vi "putHardpointStatus.vi"(8 "error in (no error)":errorcluster, 10 "TelemetryHardpointStatus":T1, 11 "M1M3SAL in":refnum<class "M1M3SAL.lvclass">) -> (0 "error out":errorcluster, 3 "M1M3SAL out":refnum<class "M1M3SAL.lvclass">)   [LabVIEW 2016, in "M1M3SupportCommunicator.lvlib" / "M1M3SAL.lvclass"]
uses:
  M1M3SAL.lvclass
  DataTypes/Topics/TelemetryHardpointStatus.ctl
  DataTypes/Topics/Parts/Timestamp.ctl
  DataTypes/MessageHeader.ctl
  DataTypes/MessageTypes.ctl
  DataTypes/MessageTopics.ctl
  M1M3SAL.lvclass/M1M3SAL.ctl
  writeU8.vi
  writeI32.vi
  writeBoolean.vi
  M1M3SupportCommunicator.lvlib
  DataTypes/Topics/M1M3SupportTopics.lvlib
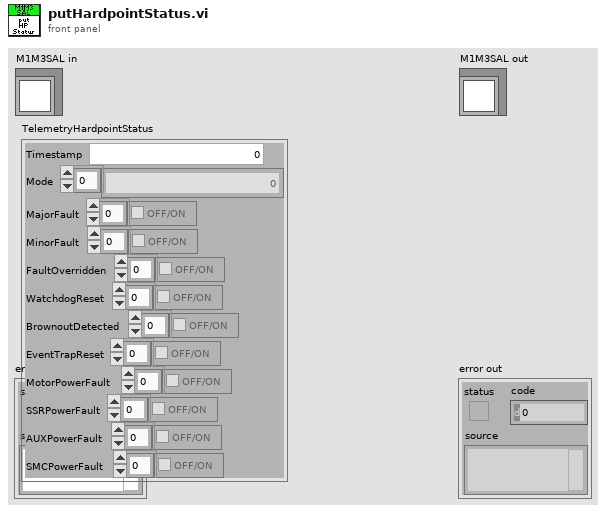
[diagram p1: front panel]
types:
  T1 = typedef "M1M3SupportTopics.lvlib/TelemetryHardpointStatus.ctl" = cluster{"Timestamp":T2, "Mode":u8[], "MajorFault":bool[], "MinorFault":bool[], "FaultOverridden":bool[], "WatchdogReset":bool[], "BrownoutDetected":bool[], "EventTrapReset":bool[], "MotorPowerFault":bool[], "SSRPowerFault":bool[], "AUXPowerFault":bool[], "SMCPowerFault":bool[]}
  T2 = typedef "M1M3SupportTopics.lvlib/Timestamp.ctl" = dbl
  T3 = typedef "M1M3SupportCommunicator.lvlib/MessageHeader.ctl" = cluster{"Type":T4, "Topic":T5, "Size":i32}
  T4 = typedef "M1M3SupportCommunicator.lvlib/MessageTypes.ctl" = enum8{"None", "PutSample", "GetNextSample", "LogEvent", "GetEvent", "IssueCommand", "CommandId", "WaitForCompletion", "AcceptCommand", "AckCommand"}
  T5 = typedef "M1M3SupportCommunicator.lvlib/MessageTopics.ctl" = enum8{"None", "ForceActuatorData", "MirrorForceData", "HardpointData", "AirData", "DynamicData", "FPGAData", "IMSData", "ForceActuatorStatus", "ElevationData", "HardpointStatus", "HardpointActuatorChase", "AirStatus", "ForceActuatorSafetyChecks", "ForceActuatorTest", "ActuatorBroadcastCounter", "StatusChecks", "CellChecks", "HardpointActuatorBreakaway", "RaiseMirrorComplete", "ILCCommunication", "ElevationAngleChecks", "DetailedState", "ServoLoops", "ForceActuatorInfo", "LowerMirrorComplete", "HardpointActuatorInfo", "SettingsApplied", "ErrorCode", "StartupChecks", "SummaryState", "SettingVersions", "ActuatorTestStatus", "AppliedSettingsMatchStart", "Enable", "EnterMaintenance", "Standby", "AbortLowerM1M3", "ApplyAberrationByForces", "ApplyAOSCorrectionByBendingModes", "ClearAOSCorrection", "Start", "RaiseM1M3", "TestForceActuator", "LowerM1M3", "ApplyAOSCorrectionByForces", "Disable", "ApplyAberationByBendingMode", "TestHardpoint", "ManipulateM1M3", "ClearAberration", "Exit", "TestAir", "AbortRaiseM1M3", "MoveHardpointActuators", "ExitMaintenance", "Shutdown"}
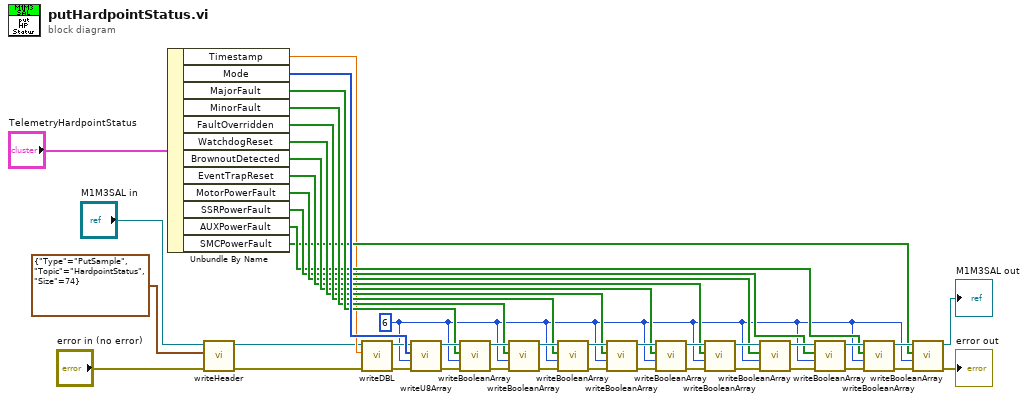
[diagram p0: block diagram]
diagram:
  w2 = 6 ("Length")
  n1 = Unbundle By Name("TelemetryHardpointStatus") -> ("Timestamp"=w9:T2, "Mode"=w20:u8[], "MajorFault"=w19:bool[], "MinorFault"=w18:bool[], "FaultOverridden"=w17:bool[], "WatchdogReset"=w16:bool[], "BrownoutDetected"=w15:bool[], "EventTrapReset"=w14:bool[], "MotorPowerFault"=w13:bool[], "SSRPowerFault"=w12:bool[], "AUXPowerFault"=w11:bool[], "SMCPowerFault"=w10:bool[])
  n2 = call "writeHeader.vi"("error in (no error)"="error in (no error)", "MessageHeader"=T3 {"Type"=enum."PutSample", "Topic"=enum."HardpointStatus", "Size"=74}, "M1M3SAL in"="M1M3SAL in") -> ("error out"=w5:errorcluster, "M1M3SAL out"=w6:refnum<class "M1M3SAL.lvclass">)  [unwired: 7 in]
  n3 = call "writeDBL.vi"("error in (no error)"=w5, "Input"=w9, "M1M3SAL in"=w6) -> ("error out"=w7:errorcluster, "M1M3SAL out"=w8:refnum<class "M1M3SAL.lvclass">)  [unwired: 7 in]
  n4 = call "writeU8Array.vi"("error in (no error)"=w7, "Length"=w2, "Input"=w20, "M1M3SAL in"=w8) -> ("error out"=w21:errorcluster, "M1M3SAL out"=w22:refnum<class "M1M3SAL.lvclass">)  [unwired: 6 in]
  n5 = call "writeBooleanArray.vi"("error in (no error)"=w21, "Length"=w2, "Input"=w19, "M1M3SAL in"=w22) -> ("error out"=w40:errorcluster, "M1M3SAL out"=w39:refnum<class "M1M3SAL.lvclass">)  [unwired: 6 in]
  n6 = call "writeBooleanArray.vi"("error in (no error)"=w40, "Length"=w2, "Input"=w18, "M1M3SAL in"=w39) -> ("error out"=w38:errorcluster, "M1M3SAL out"=w37:refnum<class "M1M3SAL.lvclass">)  [unwired: 6 in]
  n7 = call "writeBooleanArray.vi"("error in (no error)"=w38, "Length"=w2, "Input"=w17, "M1M3SAL in"=w37) -> ("error out"=w36:errorcluster, "M1M3SAL out"=w35:refnum<class "M1M3SAL.lvclass">)  [unwired: 6 in]
  n8 = call "writeBooleanArray.vi"("error in (no error)"=w36, "Length"=w2, "Input"=w16, "M1M3SAL in"=w35) -> ("error out"=w34:errorcluster, "M1M3SAL out"=w33:refnum<class "M1M3SAL.lvclass">)  [unwired: 6 in]
  n9 = call "writeBooleanArray.vi"("error in (no error)"=w34, "Length"=w2, "Input"=w15, "M1M3SAL in"=w33) -> ("error out"=w32:errorcluster, "M1M3SAL out"=w31:refnum<class "M1M3SAL.lvclass">)  [unwired: 6 in]
  n10 = call "writeBooleanArray.vi"("error in (no error)"=w32, "Length"=w2, "Input"=w14, "M1M3SAL in"=w31) -> ("error out"=w30:errorcluster, "M1M3SAL out"=w29:refnum<class "M1M3SAL.lvclass">)  [unwired: 6 in]
  n11 = call "writeBooleanArray.vi"("error in (no error)"=w30, "Length"=w2, "Input"=w13, "M1M3SAL in"=w29) -> ("error out"=w28:errorcluster, "M1M3SAL out"=w27:refnum<class "M1M3SAL.lvclass">)  [unwired: 6 in]
  n12 = call "writeBooleanArray.vi"("error in (no error)"=w28, "Length"=w2, "Input"=w12, "M1M3SAL in"=w27) -> ("error out"=w26:errorcluster, "M1M3SAL out"=w25:refnum<class "M1M3SAL.lvclass">)  [unwired: 6 in]
  n13 = call "writeBooleanArray.vi"("error in (no error)"=w26, "Length"=w2, "Input"=w11, "M1M3SAL in"=w25) -> ("error out"=w24:errorcluster, "M1M3SAL out"=w23:refnum<class "M1M3SAL.lvclass">)  [unwired: 6 in]
  n14 = call "writeBooleanArray.vi"("error in (no error)"=w24, "Length"=w2, "Input"=w10, "M1M3SAL in"=w23) -> ("error out"=→"error out":errorcluster, "M1M3SAL out"=→"M1M3SAL out":refnum<class "M1M3SAL.lvclass">)  [unwired: 6 in]
